vi "c_ctre_phoenix6_RequestControlColorFlowAnimation.vi"(0 "String 2":string, 1 "Numeric 2":u32, 2 "Numeric 3":dbl, 3 "Numeric 4":i32, 4 "Numeric 5":i32, 5 "Numeric 6":i32, 6 "Numeric 7":i32, 7 "Numeric 8":i32, 8 "Numeric 9":i32, 9 "Numeric 10":i32, 10 "Numeric 11":i32, 11 "Numeric 12":dbl) -> (20 "Numeric":i32, 21 "String":string)   [LabVIEW 2025]
uses:
  <vilib>/Rock Robotics/WPI/ThirdParty/Phoenix-LabVIEW/Controls/DriverLib.ctl
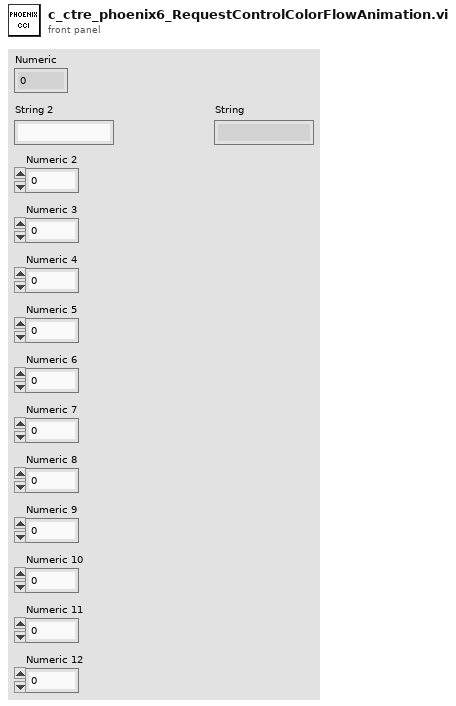
[diagram p1: front panel]
types:
  T1 = typedef "DriverLib.ctl" = path
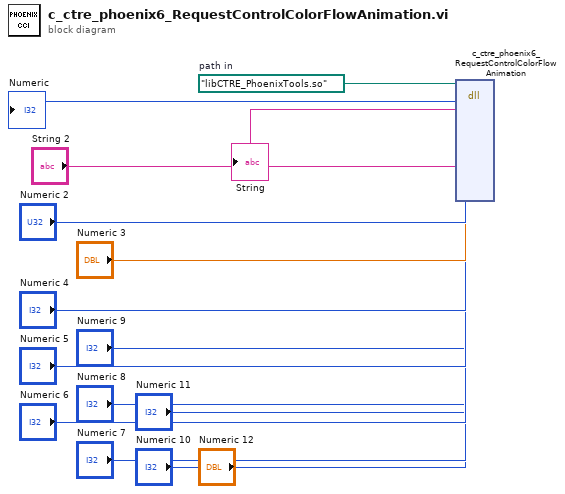
[diagram p0: block diagram]
diagram:
  w15 = T1 path "libCTRE_PhoenixTools.so"  # path in
  n1 = dll-call lib="?" fn="c_ctre_phoenix6_RequestControlColorFlowAnimation"(path in=w15, "String 2", "Numeric 2", "Numeric 3", "Numeric 4", "Numeric 5", "Numeric 6", "Numeric 7", "Numeric 8", "Numeric 9", "Numeric 10", "Numeric 11", "Numeric 12") -> (→"Numeric":i32, →"String":string)  [unwired: 13 in, 2 out]
